vi "test breakdown and compact.vi"() -> ()   [LabVIEW 2017]
uses:
  user.lib/_NEVSTOP/Communicable State Machine(CSM)/Communicable State Machine.lvlib
panel:
  in  "States 4":string="Data: Initialize\nInitialize Core Data\nEvents: Register\n\n\nUI: Initialize\nUI: Front Panel State >> Open\nMacro: Switch Active Module\n\n"
  out "States 3":string="Data: Initialize\r\nInitialize Core Data\r\nEvents: Register\r\nUI: Initialize\r\nUI: Front Panel State >> Open\r\nMacro: Switch Active Module"
  out "Multiple States 2":string[](array[string])=["Data: Initialize", "Initialize Core Data", "Events: Register", "UI: Initialize", "UI: Front Panel State >> Open", "Macro: Switch Active Module"]
  out "Multiple States":string[](array[string])=["Data: Initialize", "Initialize Core Data", "Events: Register", "UI: Initialize", "UI: Front Panel State >> Open", "Macro: Switch Active Module"]
  out "States 2":string="Data: Initialize\r\nInitialize Core Data\r\nEvents: Register\r\nUI: Initialize\r\nUI: Front Panel State >> Open\r\nMacro: Switch Active Module"
  in  "States":string="Data: Initialize\nInitialize Core Data\nEvents: Register\nUI: Initialize\nUI: Front Panel State >> Open\nMacro: Switch Active Module"
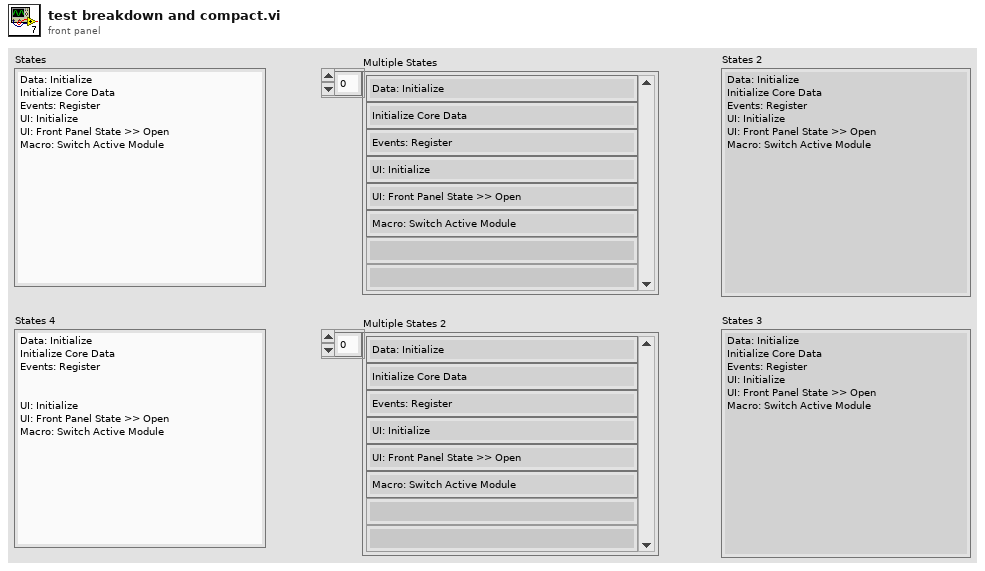
[diagram p1: front panel]
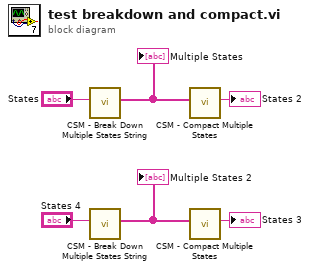
[diagram p0: block diagram]
diagram:
  n1 = call "CSM - Break Down Multiple States String.vi"("States"="States") -> ("Multiple States"=w6:string[])  [unwired: 10 in]
  "Multiple States" <- w6
  n2 = call "CSM - Break Down Multiple States String.vi"("States"="States 4") -> ("Multiple States"=w1:string[])  [unwired: 10 in]
  "Multiple States 2" <- w1
  n3 = call "CSM - Compact Multiple States.vi"("Multiple States"=w6) -> ("States"=→"States 2":string)  [unwired: 9 in]
  n4 = call "CSM - Compact Multiple States.vi"("Multiple States"=w1) -> ("States"=→"States 3":string)  [unwired: 9 in]
